vi "setTCPComunication.vi"(8 "error in (no error)":errorcluster, 10 "Settings":T1={"IP"="127.0.0.1", "port_low"=50000, "port_up"=50000, "connection_timeout "=500, "reading_timeout"=500, "writing_timeout"=500}, 11 "MonoClientCommunicator in":refnum<class "MonoClientCommunicator.lvclass">) -> (0 "error out":errorcluster, 3 "MonoClientCommunicator out":refnum<class "MonoClientCommunicator.lvclass">)   [LabVIEW 2016, in "MonoClientCommunicator.lvclass"]
uses:
  MonoClientCommunicator.lvclass
  ts_labview_tcp/tcpTypedefs/TCPSettings.ctl
  ts_labview_tcp/TCPClient/TCPClient.lvclass
  home/andres/ts_monochromator/ss_monochromator/ts_labview_tcp/TCPCommunicator/TCPCommunicator.lvclass
  ts_labview_tcp/TCPSettings/TCPSettings.lvclass
  ts_labview_tcp/TCPCommunicator/TCPCommunicator.lvclass/TCPCommunicator.ctl
  MonoClientCommunicator.lvclass/MonoClientCommunicator.ctl
  ts_labview_tcp/TCPComEvents/TCPComEvents.lvclass
  ts_labview_tcp/TCPCommunicator/TCPCommunicator.lvclass
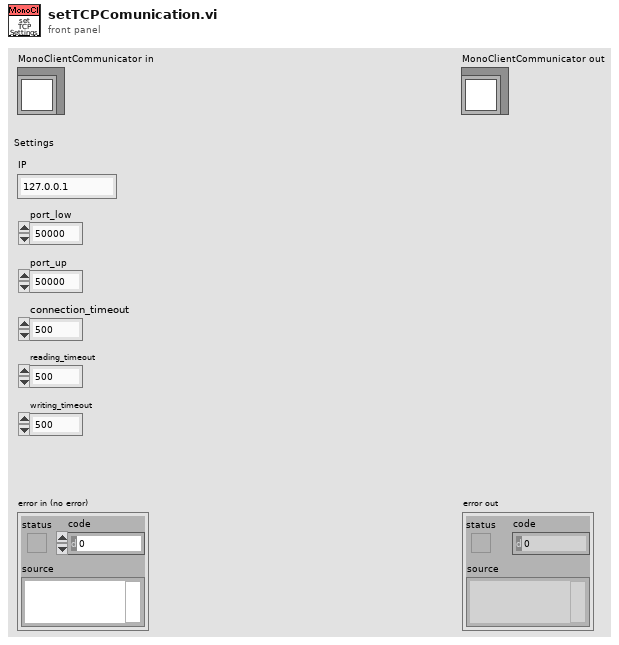
[diagram p1: front panel]
types:
  T1 = typedef "TCPSettings.ctl" = cluster{"IP":string, "port_low":u16, "port_up":u16, "connection_timeout ":i32, "reading_timeout":i32, "writing_timeout":i32}
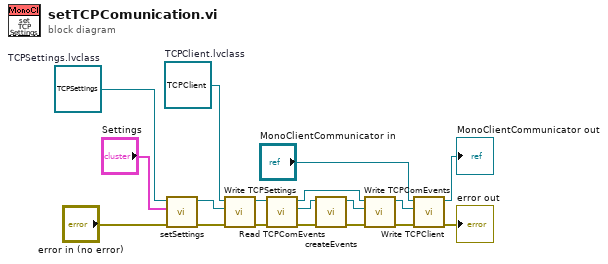
[diagram p0: block diagram]
diagram:
  w18 = refnum<class "TCPSettings.lvclass"> refnum  # TCPSettings.lvclass
  w14 = refnum<class "TCPClient.lvclass"> refnum  # TCPClient.lvclass
  n1 = call "setSettings.vi"("error in (no error)"="error in (no error)", "Settings"="Settings", "TCPSettings in"=w18) -> ("error out"=w15:errorcluster, "TCPSettings out"=w13:refnum<class "TCPSettings.lvclass">)  [unwired: 7 in]
  n2 = call-dynamic "Write TCPSettings.vi"("error in (no error)"=w15, "TCPSettings.lvclass"=w13, "TCPCommunicator in"=w14) -> ("error out"=w5:errorcluster, "TCPCommunicator out"=w6:refnum<class "TCPClient.lvclass">)  [unwired: 7 in]
  n3 = call "Read TCPComEvents.vi"("error in (no error)"=w5, "TCPCommunicator in"=w6) -> ("error out"=w4:errorcluster, "TCPComEvents.lvclass"=w10:refnum<class "TCPComEvents.lvclass">, "TCPCommunicator out"=w11:refnum<class "TCPClient.lvclass">)  [unwired: 7 in]
  n4 = call "createEvents.vi"("error in (no error)"=w4, "TCPComEvents in"=w10) -> ("error out"=w3:errorcluster, "TCPComEvents out"=w12:refnum<class "TCPComEvents.lvclass">)  [unwired: 8 in]
  n5 = call "Write TCPComEvents.vi"("error in (no error)"=w3, "TCPComEvents.lvclass"=w12, "TCPCommunicator in"=w11) -> ("error out"=w2:errorcluster, "TCPCommunicator out"=w9:refnum<class "TCPClient.lvclass">)  [unwired: 7 in]
  n6 = call "Write TCPClient.vi"("error in (no error)"=w2, "TCPClient.lvclass"=w9, "MonoClient in"="MonoClientCommunicator in") -> ("error out"=→"error out":errorcluster, "MonoClient out"=→"MonoClientCommunicator out":refnum<class "MonoClientCommunicator.lvclass">)  [unwired: 7 in]
